vi "ClosePhidget.vi"   [LabVIEW 2012]
uses:
  <instrlib>/Phidgets/Phidget Accelerometer/Phidget Accelerometer.lvlib
  <instrlib>/Phidgets/Phidget Current Input/Phidget Current Input.lvlib
  <instrlib>/Phidgets/Phidget DC Motor/Phidget DC Motor.lvlib
  <instrlib>/Phidgets/Phidget Digital Input/Phidget Digital Input.lvlib
  <instrlib>/Phidgets/Phidget Digital Output/Phidget Digital Output.lvlib
  <instrlib>/Phidgets/Phidget Encoder/Phidget Encoder.lvlib
  <instrlib>/Phidgets/Phidget Frequency Counter/Phidget Frequency Counter.lvlib
  <instrlib>/Phidgets/Phidget GPS/Phidget GPS.lvlib
  <instrlib>/Phidgets/Phidget Gyroscope/Phidget Gyroscope.lvlib
  <instrlib>/Phidgets/Phidget Humidity Sensor/Phidget Humidity Sensor.lvlib
  <instrlib>/Phidgets/Phidget IR/Phidget IR.lvlib
  <instrlib>/Phidgets/Phidget LCD/Phidget LCD.lvlib
  <instrlib>/Phidgets/Phidget Light Sensor/Phidget Light Sensor.lvlib
  <instrlib>/Phidgets/Phidget Magnetometer/Phidget Magnetometer.lvlib
  <instrlib>/Phidgets/Phidget Pressure Sensor/Phidget Pressure Sensor.lvlib
  <instrlib>/Phidgets/Phidget RC Servo/Phidget RC Servo.lvlib
  <instrlib>/Phidgets/Phidget RFID/Phidget RFID.lvlib
  <instrlib>/Phidgets/Phidget Spatial/Phidget Spatial.lvlib
  <instrlib>/Phidgets/Phidget Stepper/Phidget Stepper.lvlib
  <instrlib>/Phidgets/Phidget Temperature Sensor/Phidget Temperature Sensor.lvlib
  <instrlib>/Phidgets/Phidget Voltage Input/Phidget Voltage Input.lvlib
  <instrlib>/Phidgets/Phidget Voltage Output/Phidget Voltage Output.lvlib
  <instrlib>/Phidgets/Phidget Voltage Ratio Input/Phidget Voltage Ratio Input.lvlib
  <instrlib>/Phidgets/Phidget Capacitive Touch/Phidget Capacitive Touch.lvlib
  <instrlib>/Phidgets/Phidget PH Sensor/Phidget PH Sensor.lvlib
  <instrlib>/Phidgets/Phidget Distance Sensor/Phidget Distance Sensor.lvlib
  <instrlib>/Phidgets/Phidget Sound Sensor/Phidget Sound Sensor.lvlib
  <instrlib>/Phidgets/Phidget Resistance Input/Phidget Resistance Input.lvlib
  <instrlib>/Phidgets/Phidget Power Guard/Phidget Power Guard.lvlib
  <instrlib>/Phidgets/Phidget Motor Position Controller/Phidget Motor Position Controller.lvlib
  <instrlib>/Phidgets/Phidget BLDC Motor/Phidget BLDC Motor.lvlib
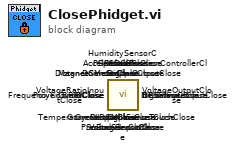
[diagram p0: block diagram]
diagram:
  n1 = call <instrlib>:"BLDCMotorClose.vi"() -> ()  [unwired: 11 in, 1 out]
  n2 = call <instrlib>:"MotorPositionControllerClose.vi"() -> ()  [unwired: 11 in, 1 out]
  n3 = call <instrlib>:"PowerGuardClose.vi"() -> ()  [unwired: 11 in, 1 out]
  n4 = call <instrlib>:"ResistanceInputClose.vi"() -> ()  [unwired: 11 in, 1 out]
  n5 = call <instrlib>:"SoundSensorClose.vi"() -> ()  [unwired: 11 in, 1 out]
  n6 = call <instrlib>:"DistanceSensorClose.vi"() -> ()  [unwired: 11 in, 1 out]
  n7 = call <instrlib>:"PHSensorClose.vi"() -> ()  [unwired: 11 in, 1 out]
  n8 = call <instrlib>:"CapacitiveTouchClose.vi"() -> ()  [unwired: 11 in, 1 out]
  n9 = call <instrlib>:"VoltageRatioInputClose.vi"() -> ()  [unwired: 11 in, 1 out]
  n10 = call <instrlib>:"VoltageOutputClose.vi"() -> ()  [unwired: 11 in, 1 out]
  n11 = call <instrlib>:"VoltageInputClose.vi"() -> ()  [unwired: 11 in, 1 out]
  n12 = call <instrlib>:"TemperatureSensorClose.vi"() -> ()  [unwired: 11 in, 1 out]
  n13 = call <instrlib>:"StepperClose.vi"() -> ()  [unwired: 11 in, 1 out]
  n14 = call <instrlib>:"SpatialClose.vi"() -> ()  [unwired: 11 in, 1 out]
  n15 = call <instrlib>:"RFIDClose.vi"() -> ()  [unwired: 11 in, 1 out]
  n16 = call <instrlib>:"RCServoClose.vi"() -> ()  [unwired: 11 in, 1 out]
  n17 = call <instrlib>:"PressureSensorClose.vi"() -> ()  [unwired: 11 in, 1 out]
  n18 = call <instrlib>:"MagnetometerClose.vi"() -> ()  [unwired: 11 in, 1 out]
  n19 = call <instrlib>:"LightSensorClose.vi"() -> ()  [unwired: 11 in, 1 out]
  n20 = call <instrlib>:"LCDClose.vi"() -> ()  [unwired: 11 in, 1 out]
  n21 = call <instrlib>:"IRClose.vi"() -> ()  [unwired: 11 in, 1 out]
  n22 = call <instrlib>:"HumiditySensorClose.vi"() -> ()  [unwired: 11 in, 1 out]
  n23 = call <instrlib>:"GyroscopeClose.vi"() -> ()  [unwired: 11 in, 1 out]
  n24 = call <instrlib>:"GPSClose.vi"() -> ()  [unwired: 11 in, 1 out]
  n25 = call <instrlib>:"FrequencyCounterClose.vi"() -> ()  [unwired: 11 in, 1 out]
  n26 = call <instrlib>:"EncoderClose.vi"() -> ()  [unwired: 11 in, 1 out]
  n27 = call <instrlib>:"DigitalOutputClose.vi"() -> ()  [unwired: 11 in, 1 out]
  n28 = call <instrlib>:"DigitalInputClose.vi"() -> ()  [unwired: 11 in, 1 out]
  n29 = call <instrlib>:"DCMotorClose.vi"() -> ()  [unwired: 11 in, 1 out]
  n30 = call <instrlib>:"CurrentInputClose.vi"() -> ()  [unwired: 11 in, 1 out]
  n31 = call <instrlib>:"AccelerometerClose.vi"() -> ()  [unwired: 11 in, 1 out]
